vi "Divide Polynomials (CDB).vi"(8 "threshold type":T1 items=["Absolute Value", "Relative Value"], 9 "threshold":dbl, 10 "Q(x)":cdb[](array[numeric]), 11 "P(x)":cdb[](array[numeric])) -> (0 "error":i32, 2 "Remainder":cdb[](array[numeric]), 3 "P(x)/Q(x)":cdb[](array[numeric]))   [LabVIEW 2020, in "NI_AALPro.lvlib"]
doc: "Divides polynomial <B>P(x)</B> by polynomial <B>Q(x)</B>. The data types you wire to the <B>P(x)</B> and <B>Q(x)</B> inputs determine the polymorphic instance to use."
uses:
  <vilib>/Analysis/NI_AALPro.lvlib
  <vilib>/Analysis/polynomials.llb/Remove Zero Threshold Type.ctl
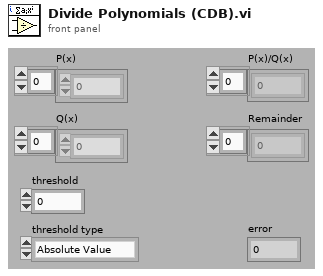
[diagram p1: front panel]
types:
  T1 = typedef "NI_AALPro.lvlib/Remove Zero Threshold Type.ctl" = u16
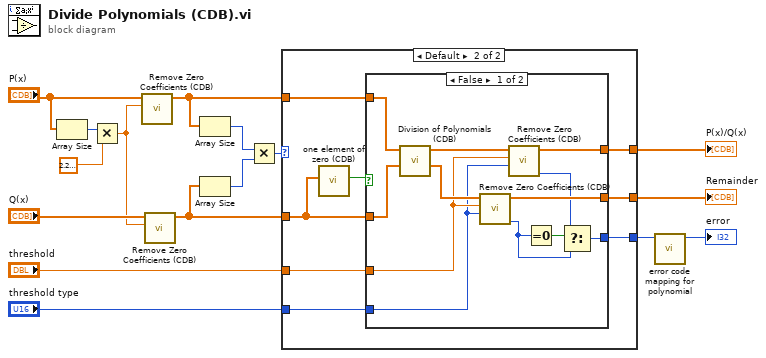
[diagram p0: block diagram]
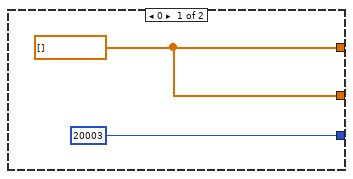
[diagram p2: hidden frame]
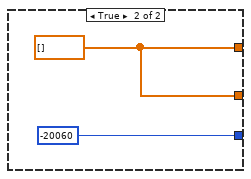
[diagram p3: hidden frame]
diagram:
  n1 = Array Size(array="P(x)") -> (size(s)=w16:i32)
  n2 = Multiply(x=w16, y=2.220446049250313e-16) -> (x*y=w9:dbl)
  n3 = call <vilib>:"Remove Zero Coefficients (CDB).vi"("threshold"=w9, "P(x) In"="P(x)") -> ("P(x) Out"=w12:cdb[])  [unwired: 7 in, 2 out]
  n4 = call <vilib>:"Remove Zero Coefficients (CDB).vi"("threshold"=w9, "P(x) In"="Q(x)") -> ("P(x) Out"=w8:cdb[])  [unwired: 7 in, 2 out]
  n5 = Array Size(array=w12) -> (size(s)=w14:i32)
  n6 = Array Size(array=w8) -> (size(s)=w13:i32)
  n7 = Multiply(x=w14, y=w13) -> (x*y=w11:i32)
  n8 = case shown="Default" w11 {
    tunnel: w8 -> [_ w22]
    tunnel: w12 -> [_ w26]
    tunnel: [w18 w25] -> w7
    tunnel: [w18 w24] -> w6
    tunnel: [20003 ("empty array") w23] -> w5
    tunnel: "threshold" -> [_ w20]
    tunnel: "threshold type" -> [_ w19]
    frame 0 {
      w18 = cdb[] []
    }
    frame Default {
      n9 = call <vilib>:"one element of zero (CDB).vi"("Array in"=w22) -> ("equal [0]?"=w21:bool)  [unwired: 10 in]
      n10 = case shown="False" w21 {
        tunnel: w22 -> [w37 _]
        tunnel: w26 -> [w38 _]
        tunnel: [w35 w40] -> w25
        tunnel: [w34 w40] -> w24
        tunnel: [w29 -20060 ("divide by zero")] -> w23
        tunnel: w20 -> [w28 _]
        tunnel: w19 -> [w27 _]
        frame False {
          n11 = call <vilib>:"Division of Polynomials (CDB).vi"("q"=w37, "p"=w38) -> ("rest"=w33:cdb[], "p/q"=w36:cdb[])  [unwired: 8 in]
          n12 = call <vilib>:"Remove Zero Coefficients (CDB).vi"("threshold type"=w27, "threshold"=w28, "P(x) In"=w33) -> ("error"=w30:i32, "P(x) Out"=w34:cdb[])  [unwired: 6 in, 1 out]
          n13 = call <vilib>:"Remove Zero Coefficients (CDB).vi"("threshold type"=w27, "threshold"=w28, "P(x) In"=w36) -> ("error"=w31:i32, "P(x) Out"=w35:cdb[])  [unwired: 6 in, 1 out]
          n14 = Equal To 0?(x=w30) -> (x = 0?=w32:bool)
          n15 = Select(t=w31, s=w32, f=w30) -> (s? t:f=w29:i32)
        }
        frame True {
          w40 = cdb[] []
        }
      }
    }
  }
  "Remainder" <- w6
  "P(x)/Q(x)" <- w7
  n16 = call <vilib>:"error code mapping for polynomial.vi"("error in"=w5) -> ("error out"=→"error":i32)  [unwired: 10 in]
